vi "test_color.vi"() -> ()   [LabVIEW 2013]
panel:
  out "Numeric 2":dbl
  in  "limit sup":dbl(knob) scale=0.0..10.0
  in  "limit inf":dbl(knob) scale=0.0..10.0
  in  "stop":bool
  in  "signal":dbl(knob) scale=0.0..10.0
  out "Numeric":dbl
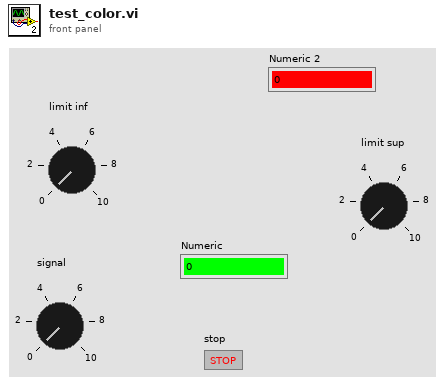
[diagram p1: front panel]
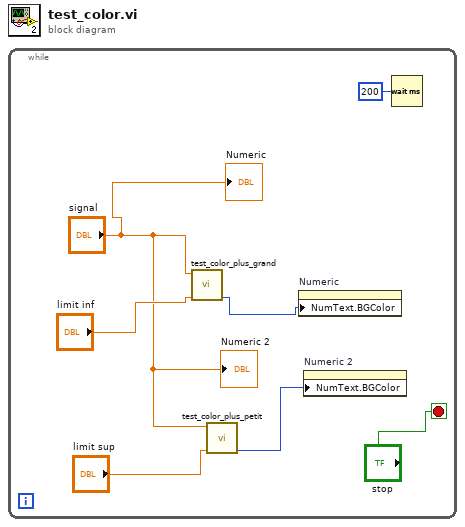
[diagram p0: block diagram]
diagram:
  n1 = while {
    stop <- "stop" stop-if-true
    n2 = call "test_color_plus_grand.vi"("limite inférieure"="limit inf", "signal"="signal") -> ("result color"=w5:u32)  [unwired: 9 in]
    n3 = call "test_color_plus_petit.vi"("limite supérieure"="limit sup", "signal"="signal") -> ("result color"=w1:u32)  [unwired: 9 in]
    n4 = property on="Numeric" class="DigNum (strict)"("NumText.BGColor"=w5) -> ()  [unwired: 2 in, 2 out]
    n5 = property on="Numeric 2" class="DigNum (strict)"("NumText.BGColor"=w1) -> ()  [unwired: 2 in, 2 out]
    n6 = Wait (ms)(milliseconds to wait=u32 200) -> ()  [unwired: 1 out]
    "Numeric" <- "signal"
    "Numeric 2" <- "signal"
  }
